vi "Read String Length.vi"(11 "RandomStringGenerator in":refnum<class "RandomStringGenerator.lvclass">) -> (2 "String Length":u32, 3 "RandomStringGenerator out":refnum<class "RandomStringGenerator.lvclass">)   [LabVIEW 2014, in "RandomStringGenerator.lvclass"]
uses:
  RandomStringGenerator.lvclass
  RandomStringGenerator.lvclass/RandomStringGenerator.ctl
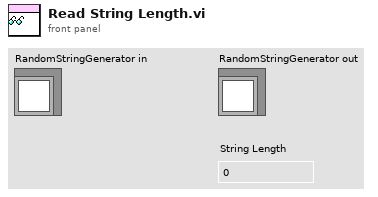
[diagram p1: front panel]
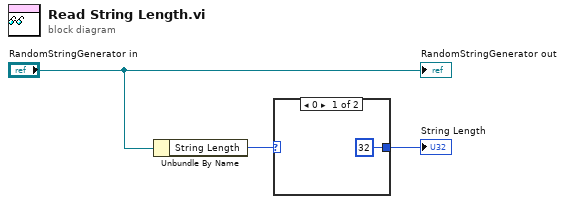
[diagram p0: block diagram]
diagram:
  n1 = Unbundle By Name("RandomStringGenerator in") -> ("String Length"=w2:u32)
  n2 = case shown="0" w2 {
    selector: w2 -> [_ w5]
    tunnel: [u32 32 ("String Length") w5] -> w1
    frame 0 {
    }
    frame Default {
    }
  }
  "String Length" <- w1
  "RandomStringGenerator out" <- "RandomStringGenerator in"
